vi "Get ErrorCluster.vi"(8 "error in (no error)":errorcluster, 11 "ErrorMessage in":refnum<class "ErrorMessage.lvclass">) -> (0 "error out":errorcluster, 2 "ErrorCluster":errorcluster, 3 "ErrorMessage out":refnum<class "ErrorMessage.lvclass">)   [LabVIEW 2009, in "LapDog.Messaging.v2.lvlib" / "ErrorMessage.lvclass"]
doc: "Returns the error cluster contained in the error message.\n\nThis method executes regardless of the error in state."
uses:
  ErrorMessage.lvclass
  ErrorMessage.lvclass/ErrorMessage.ctl
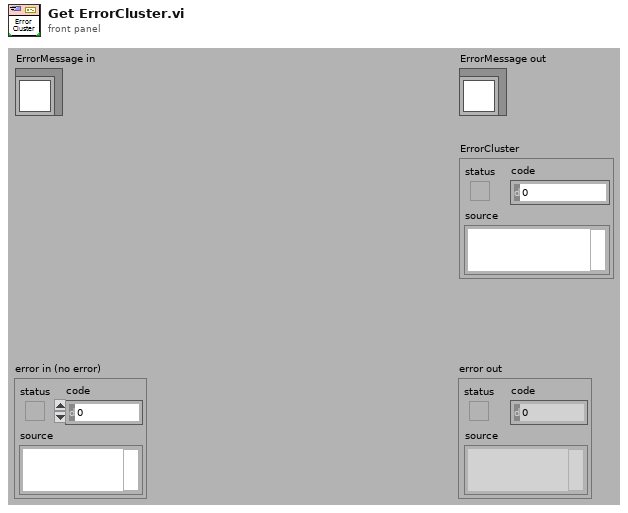
[diagram p1: front panel]
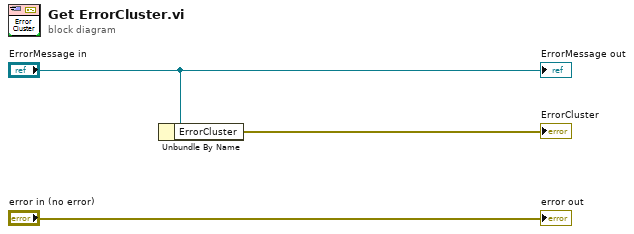
[diagram p0: block diagram]
diagram:
  n1 = Unbundle By Name("ErrorMessage in") -> ("ErrorCluster"=→"ErrorCluster":errorcluster)
  "error out" <- "error in (no error)"
  "ErrorMessage out" <- "ErrorMessage in"
